vi "setTimes.vi"(8 "error in (no error)":errorcluster, 10 "times":dbl[](array[numeric]), 11 "DeviceData.lvclass in":refnum<class "DeviceData.lvclass">) -> (0 "error out":errorcluster, 3 "DeviceData.lvclass out":refnum<class "DeviceData.lvclass">)   [LabVIEW 2011, in "DataMappers.lvlib" / "DeviceData.lvclass"]
uses:
  DeviceData.lvclass
  DeviceData.lvclass/DeviceData.ctl
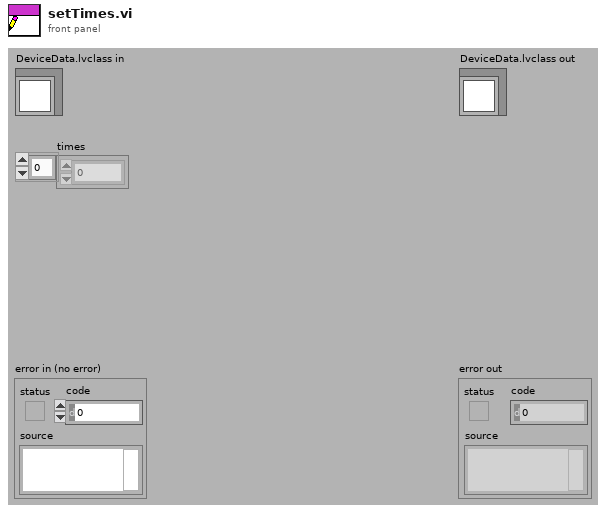
[diagram p1: front panel]
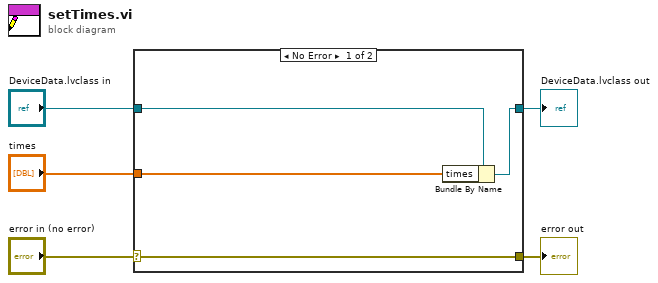
[diagram p0: block diagram]
diagram:
  n1 = case shown="No Error" "error in (no error)" {
    selector: "error in (no error)" -> [w9 w10]
    tunnel: [w9 w10] -> w4
    tunnel: [w7 w11] -> w2
    tunnel: "DeviceData.lvclass in" -> [w8 w11]
    tunnel: "times" -> [w6 _]
    frame No Error {
      n2 = Bundle By Name(cluster=w8, "times"=w6) -> (w7:refnum<class "DeviceData.lvclass">)
    }
    frame Error {
    }
  }
  "error out" <- w4
  "DeviceData.lvclass out" <- w2
